vi "GetPosition.vi"(5 "Axis":string="Horizontal Rotator", 6 "error in (no error)":errorcluster, 7 "Instrument Ref In":refnum<k24>) -> (0 "GetPosition Error":i32, 1 "Position":dbl, 2 "error out":errorcluster, 3 "Instrument Ref Out":refnum<k24>)   [LabVIEW 2016]
uses:
  C:/user/repos/levylab_inst_ppms2/lvsrc/QDInstrument_LabView/QDInstrument.dll
  QDInstrument.dll
panel:
  out "GetPosition\nStatus":i32(ring) items=["PositionUnknown", "AtTarget", "Unused2", "Unused3", "Unused4", "Moving", "Unused6", "Unused7", "AtLimitSwitch", "AtIndexSwitch", "Unused10", "Unused11", "Unused12", "Unused13", "Unused14", "PositionFailure"]
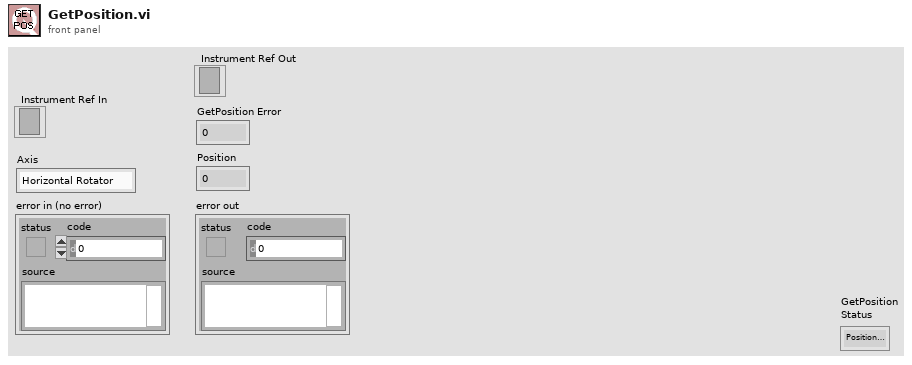
[diagram p1: front panel]
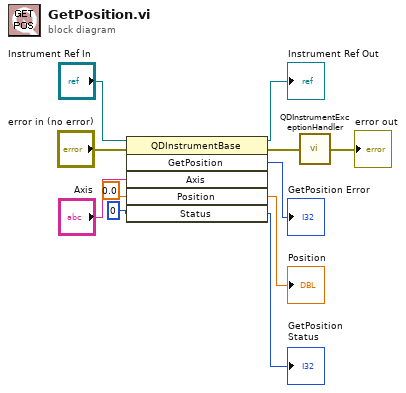
[diagram p0: block diagram]
diagram:
  n1 = invoke class="QDInstrumentBase" method="GetPosition"(reference="Instrument Ref In", error in="error in (no error)", "Axis"="Axis", "Position"=0.0 ("Temperature"), "Status"=0) -> (reference out=→"Instrument Ref Out":refnum<k24>, error out=w7:errorcluster, "GetPosition"=→"GetPosition Error":i32, "Position"=→"Position":dbl, "Status"=→"GetPosition\nStatus":i32)  [unwired: 1 in, 1 out]
  n2 = call "QDInstrumentExceptionHandler.vi"("Error in"=w7) -> ("Error out"=→"error out":errorcluster)
